vi "Handling AI scada.vi"(8 "error in":errorcluster, 9 "color_schema":i32[](array[numeric])=[0], 10 "AI_reorder_table":i32[](array[numeric]), 11 "OPC UA.Client refnum":T2) -> (0 "error":errorcluster, 1 "AIALRState":errorcluster[](array[cluster]), 2 "AIState":T1[](array[typedef]), 3 "AI":dbl[](array[numeric]), 4 "connect":bool)   [LabVIEW 2019, in "Inputs.lvlib"]
uses:
  Inputs.lvlib
  <vilib>/OPCUA/controls/OPC UA Client Refnum.ctl
  Ctl/Parameter State.ctl
  <vilib>/OPCUA/controls/NodeIds.ctl
  <vilib>/OPCUA/controls/NodeId.ctl
  <vilib>/OPCUA/client/Multiple Read Double Array.vi
  <vilib>/OPCUA/client/Multiple Read Int32 Array.vi
  <vilib>/OPCUA/NI OPC UA Client.lvlib
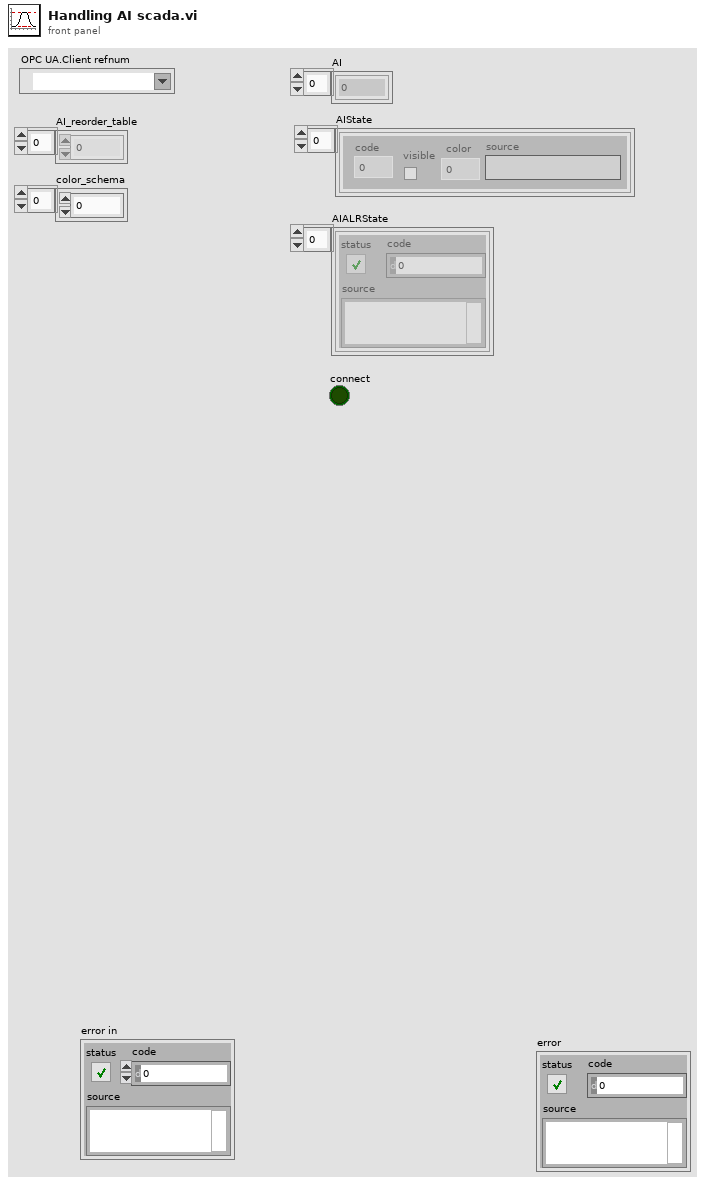
[diagram p1: front panel]
types:
  T1 = typedef "Inputs.lvlib/Parameter State.ctl" = cluster{"code":i32, "visible":bool, "color":u32, "source":string}
  T2 = typedef "OPC UA Client Refnum.ctl" = refnum<k21>
  T3 = typedef "NodeIds.ctl" = T4[]
  T4 = typedef "NodeId.ctl" = string
  T5 = typedef "OPC UA StatusCode.ctl" = u32
  T6 = cluster{"node ID":T4, "values ":dbl[], "timestamp":timestamp, "status":T5}[]
  T7 = cluster{"node ID":T4, "values ":i32[], "timestamp":timestamp, "status":T5}[]
  T8 = cluster{"node ID":T4, "values ":dbl[], "timestamp":timestamp, "status":T5}
  T9 = cluster{"node ID":T4, "values ":i32[], "timestamp":timestamp, "status":T5}
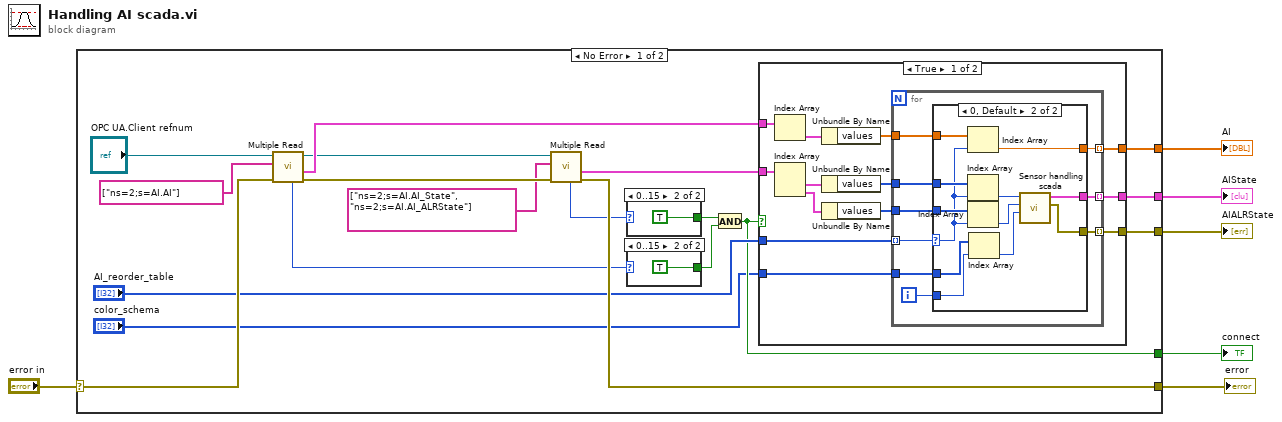
[diagram p0: block diagram]
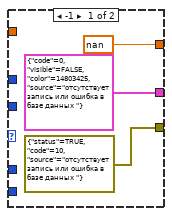
[diagram p4: hidden frame]
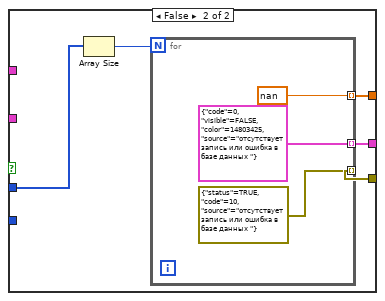
[diagram p5: hidden frame]
diagram:
  n1 = case shown="No Error" "error in" {
    selector: "error in" -> [w25 w73]
    tunnel: [w24 w73] -> w5
    tunnel: [w11 _] -> w4
    tunnel: [w10 _] -> w3
    tunnel: [w9 _] -> w2
    tunnel: [w8 _] -> w1
    frame No Error {
      n2 = call-poly <vilib>:"Multiple Read.vi"("error in (no error)"=w25, "node IDs"=T3 ["ns=2;s=AI.AI"] ("OPC UA.node IDs"), "OPC UA client refnum in"="OPC UA.Client refnum") -> ("error out"=w20:errorcluster, "results"=w23:T6, "OPC UA client refnum out"=w21:T2, "service status"=w18:T5)  [unwired: 5 in]
      n3 = call-poly <vilib>:"Multiple Read.vi"("error in (no error)"=w20, "node IDs"=T3 ["ns=2;s=AI.AI_State", "ns=2;s=AI.AI_ALRState"] ("OPC UA.node IDs"), "OPC UA client refnum in"=w21) -> ("error out"=w24:errorcluster, "results"=w14:T7, "service status"=w17:T5)  [unwired: 5 in, 1 out]
      n4 = case shown="0..15" w17 {
        tunnel: [_ TRUE] -> w16
        frame 16.., Default {
        }
        frame 0..15 {
        }
      }
      n5 = case shown="0..15" w18 {
        tunnel: [_ TRUE] -> w15
        frame 16.., Default {
        }
        frame 0..15 {
        }
      }
      n6 = And(x=w16, y=w15) -> (x .and. y?=w8:bool)
      n7 = case shown="True" w8 {
        tunnel: w23 -> [w39 _]
        tunnel: w14 -> [w38 _]
        tunnel: "AI_reorder_table" -> [w33 w68]
        tunnel: [w31 w67] -> w9
        tunnel: [w30 w66] -> w10
        tunnel: [w29 w65] -> w11
        tunnel: "color_schema" -> [w28 _]
        frame True {
          n8 = Index Array(array=w39) -> (element=w40:T8)  [unwired: 1 in]
          n9 = Index Array(array=w38) -> (element #1=w37:T9, element #2=w35:T9)  [unwired: 2 in]
          n10 = Unbundle By Name(w40) -> ("values"=w36:dbl[])
          n11 = Unbundle By Name(w37) -> ("values"=w34:i32[])
          n12 = Unbundle By Name(w35) -> ("values"=w32:i32[])
          n13 = for {
            tunnel: w36 -> [w49]
            tunnel: w33 -> [w45] mode=indexing
            tunnel: [w48] -> w31 mode=indexing
            tunnel: w32 -> [w47]
            tunnel: [w46] -> w30 mode=indexing
            tunnel: w34 -> [w44]
            tunnel: [w43] -> w29 mode=indexing
            tunnel: w28 -> [w42]
            i -> [w41]
            n14 = case shown="0, Default" w45 {
              selector: w45 -> [_ w56]
              tunnel: w49 -> [_ w64]
              tunnel: [nan ("PV") w63] -> w48
              tunnel: w47 -> [_ w62]
              tunnel: [T1 {"code"=0, "visible"=FALSE, "color"=14803425, "source"="отсутствует запись или ошибка в базе данных "} ("STATE") w58] -> w46
              tunnel: w44 -> [_ w61]
              tunnel: [errorcluster {"status"=TRUE, "code"=10, "source"="отсутствует запись или ошибка в базе данных "} ("ALRSTATE") w57] -> w43
              tunnel: w42 -> [_ w55]
              tunnel: w41 -> [_ w53]
              frame -1 {
              }
              frame 0, Default {
                n15 = Index Array(array=w64, index=w56) -> (element=w63:dbl)
                n16 = Index Array(array=w61, index=w56) -> (element=w60:i32)
                n17 = Index Array(array=w62, index=w56) -> (element=w59:i32)
                n18 = Index Array(array=w55, index=w53) -> (element=w54:i32)
                n19 = call "Sensor handling scada.vi"("color schema"=w54, "AI_ALRState"=w59, "AI_State"=w60) -> ("ALRSTATE"=w57:errorcluster, "STATE"=w58:T1)  [unwired: 7 in]
              }
            }
          }
        }
        frame False {
          n20 = Array Size(array=w68) -> (size(s)=w69:i32)
          n21 = for {
            N: w69 -> [_]
            tunnel: [nan ("PV")] -> w67 mode=indexing
            tunnel: [T1 {"code"=0, "visible"=FALSE, "color"=14803425, "source"="отсутствует запись или ошибка в базе данных "} ("STATE")] -> w66 mode=indexing
            tunnel: [errorcluster {"status"=TRUE, "code"=10, "source"="отсутствует запись или ошибка в базе данных "} ("ALRSTATE")] -> w65 mode=indexing
          }
        }
      }
    }
    frame Error {
    }
  }
  "error" <- w5
  "AI" <- w2
  "AIState" <- w3
  "AIALRState" <- w4
  "connect" <- w1
